vi "Peak Detector.vi"(4 "end of data (T)":bool=TRUE, 6 "initialize (T)":bool=TRUE, 8 "peaks/valleys":enum32{"Peaks", "Valleys"}(ring), 9 "width":i32=3 min=3, 10 "threshold":dbl format="%0.2f", 11 "X":dbl[](array[numeric])) -> (0 "error":i32, 1 "2nd Derivatives":dbl[](array[numeric]), 2 "Amplitudes":dbl[](array[numeric]), 3 "Locations":dbl[](array[numeric]), 5 "# found":i32)   [LabVIEW 2020, in "NI_AAL_SigProc.lvlib"]
doc: "Finds the location, amplitude, and second derivative of peaks or valleys in the input signal."
uses:
  <vilib>/Analysis/NI_AAL_SigProc.lvlib
  <resource>/lvanlys.dll
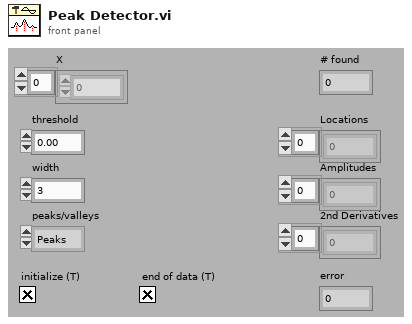
[diagram p1: front panel]
types:
  T1 = cluster{"Span":i32, "Index":i32, "NHistoryPts":i32, "Len":i32, "PrevSign":i32, "unused":i32, "RinvQt (pointer)":u32, "FitBuffer (pointer)":u32, "History (pointer)":u32, "PrevCoeff (pointer)":u32, "Data (pointer)":u32, "slack for RinvQt":u32, "slack for FitBuffer":u32, "slack for History":u32, "slack for PrevCoeff":u32, "slack for Data":u32}
  T2 = cluster{"Array Constant":dbl[], "threshold":dbl, "Span":i32, "peaks/valleys":enum32{"Peaks", "Valleys"}, "Array Constant":dbl[], "Array Constant":dbl[], "Array Constant":dbl[], i32, i32}
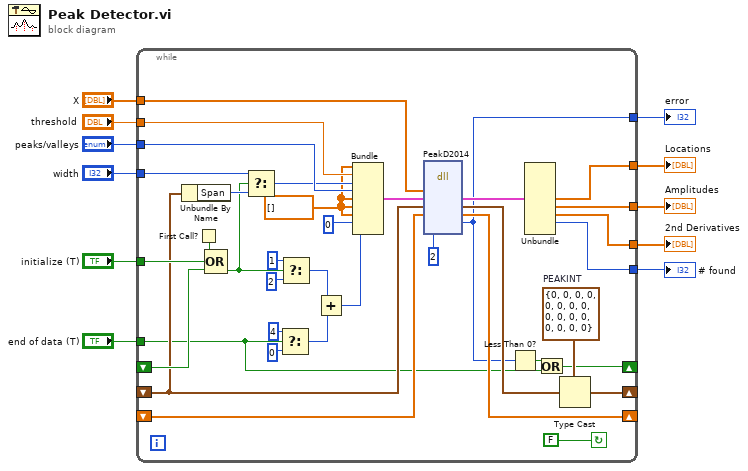
[diagram p0: block diagram]
diagram:
  n1 = while {
    shift-left: _ -> [w35]
    shift-right: [w25] -> _
    shift-left: _ -> [w31]
    shift-right: [w26] -> _
    shift-right: [w16] -> _
    shift-left: _ -> [w38]
    tunnel: "X" -> [w13]
    tunnel: "threshold" -> [w34]
    tunnel: "width" -> [w27]
    tunnel: "peaks/valleys" -> [w33]
    tunnel: "end of data (T)" -> [w17]
    tunnel: "initialize (T)" -> [w32]
    tunnel: [w14] -> w5
    tunnel: [w24] -> w4
    tunnel: [w23] -> w3
    tunnel: [w22] -> w2
    tunnel: [w21] -> w1
    stop <- FALSE continue-if-true
    w39 = T1 {"Span"=0, "Index"=0, "NHistoryPts"=0, "Len"=0, "PrevSign"=0, "unused"=0, "RinvQt (pointer)"=0, "FitBuffer (pointer)"=0, "History (pointer)"=0, "PrevCoeff (pointer)"=0, "Data (pointer)"=0, "slack for RinvQt"=0, "slack for FitBuffer"=0, "slack for History"=0, "slack for PrevCoeff"=0, "slack for Data"=0}  # PEAKINT
    w12 = dbl[] [] ("Array Constant")
    n2 = Unbundle By Name(w31) -> ("Span"=w30:i32)
    n3 = First Call?() -> (First Call?: T/F=w37:bool)
    n4 = Compound Arithmetic op=OR(w37, w32, w38) -> (w29:bool)
    n5 = Select(t=w27, s=w29, f=w30) -> (s? t:f=w28:i32)
    n6 = Select(t=4, s=w17, f=0) -> (s? t:f=w19:i32)
    n7 = Select(t=1, s=w29, f=2) -> (s? t:f=w20:i32)
    n8 = Add(x=w20, y=w19) -> (x+y=w43:i32)
    n9 = Bundle("Array Constant"=w12, "threshold"=w34, "Span"=w28, "peaks/valleys"=w33, "Array Constant"=w12, "Array Constant"=w12, "Array Constant"=w12, 0, w43) -> (w36:T2)  [unwired: 1 out]
    n10 = dll-call lib="e:/builds/penguin/labview/branches/2020/dev/dist/resource/lvanlys.*" fn="PeakD2014"("xH"=w13, "PeakApp"=w36, "pPEAKINT"=w31, "SavedData"=w35, "version"=2) -> ("PeakApp"=w42:T2, "pPEAKINT"=w40:T1, "SavedData"=w25:dbl[], "pErr"=w14:i32)  [unwired: 3 in, 6 out]
    n11 = Less Than 0?(x=w14) -> (x < 0?=w15:bool)
    n12 = Unbundle(w42) -> ("Array Constant"=w24:dbl[], "Array Constant"=w23:dbl[], "Array Constant"=w22:dbl[], w21:i32)  [unwired: 5 out]
    n13 = Or(x=w15, y=w17) -> (x .or. y?=w16:bool)
    n14 = Type Cast(type=w39, x=w40) -> (*(type *) &x=w26:T1)
  }
  "Locations" <- w4
  "Amplitudes" <- w3
  "2nd Derivatives" <- w2
  "error" <- w5
  "# found" <- w1
